vi "cameraSetup.vi"() -> ()   [LabVIEW 2024]
uses:
  <vilib>/userDefined/High Color/IMAQdx.ctl
  <vilib>/Python/Open Venv Python Session.vi
  <vilib>/vision/driver/NI_Vision_Acquisition_Software.lvlib
panel:
  out "Tracking_Err(m)":dbl=4862130.802033398
  in  "Ld(m)":dbl=5.0 format="%#_13g"
  out "GPS_Steer_CMD(Deg)":dbl=2.9943056426975447
  out "Lane":T1(graph)
  out "Third_Lane_X":dbl[](array[numeric])
  out "Third_Lane_Y":dbl[](array[numeric])
  out "Second_Lane_X":dbl[](array[numeric])
  out "Second_Lane_Y":dbl[](array[numeric])
  out "First_Lane_Y":dbl[](array[numeric])
  out "First_Lane_X":dbl[](array[numeric])
  out "ImageString":string
  out "error out":errorcluster
  out "Image":T2(plugin-control)
  in  "Test":bool=TRUE
  in  "Cam No.":T3
  out "Python Loop Process Time":u32=101
  out "Image2Array LoopTime":u32=101
  in  "stop":bool
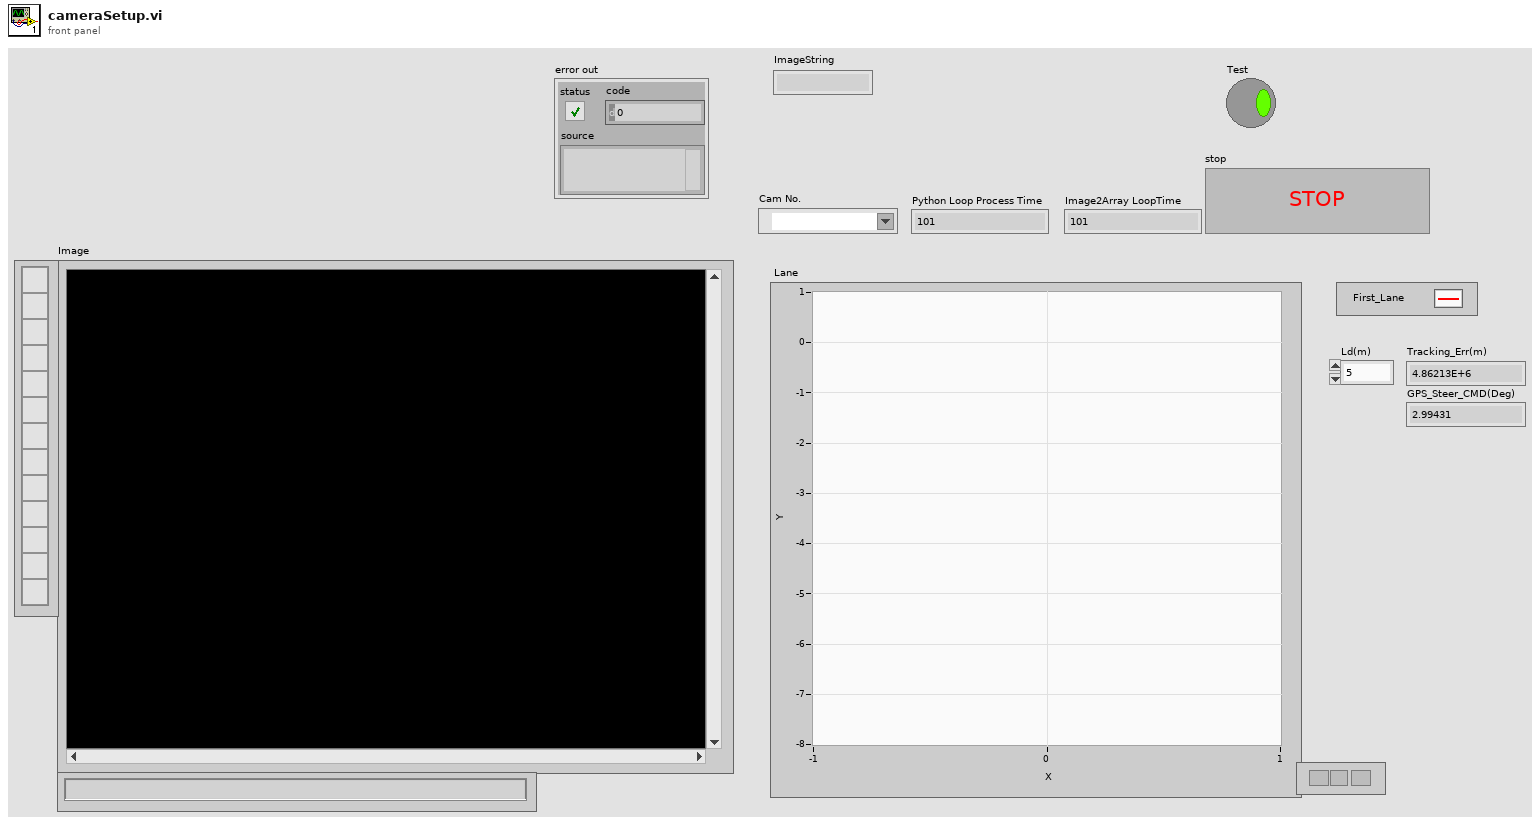
[diagram p1: front panel]
types:
  T1 = cluster{"Third_Lane_X":dbl[], "Third_Lane_Y":dbl[]}[]
  T2 = typedef "IMAQ Image.ctl" = refnum<image>
  T3 = typedef "IMAQdx.ctl" = refnum<k21>
  T4 = cluster{"First_Lane_X":dbl[], "First_Lane_Y":dbl[]}
  T5 = cluster{"Second_Lane_X":dbl[], "Second_Lane_Y":dbl[]}
  T6 = cluster{"Third_Lane_X":dbl[], "Third_Lane_Y":dbl[]}
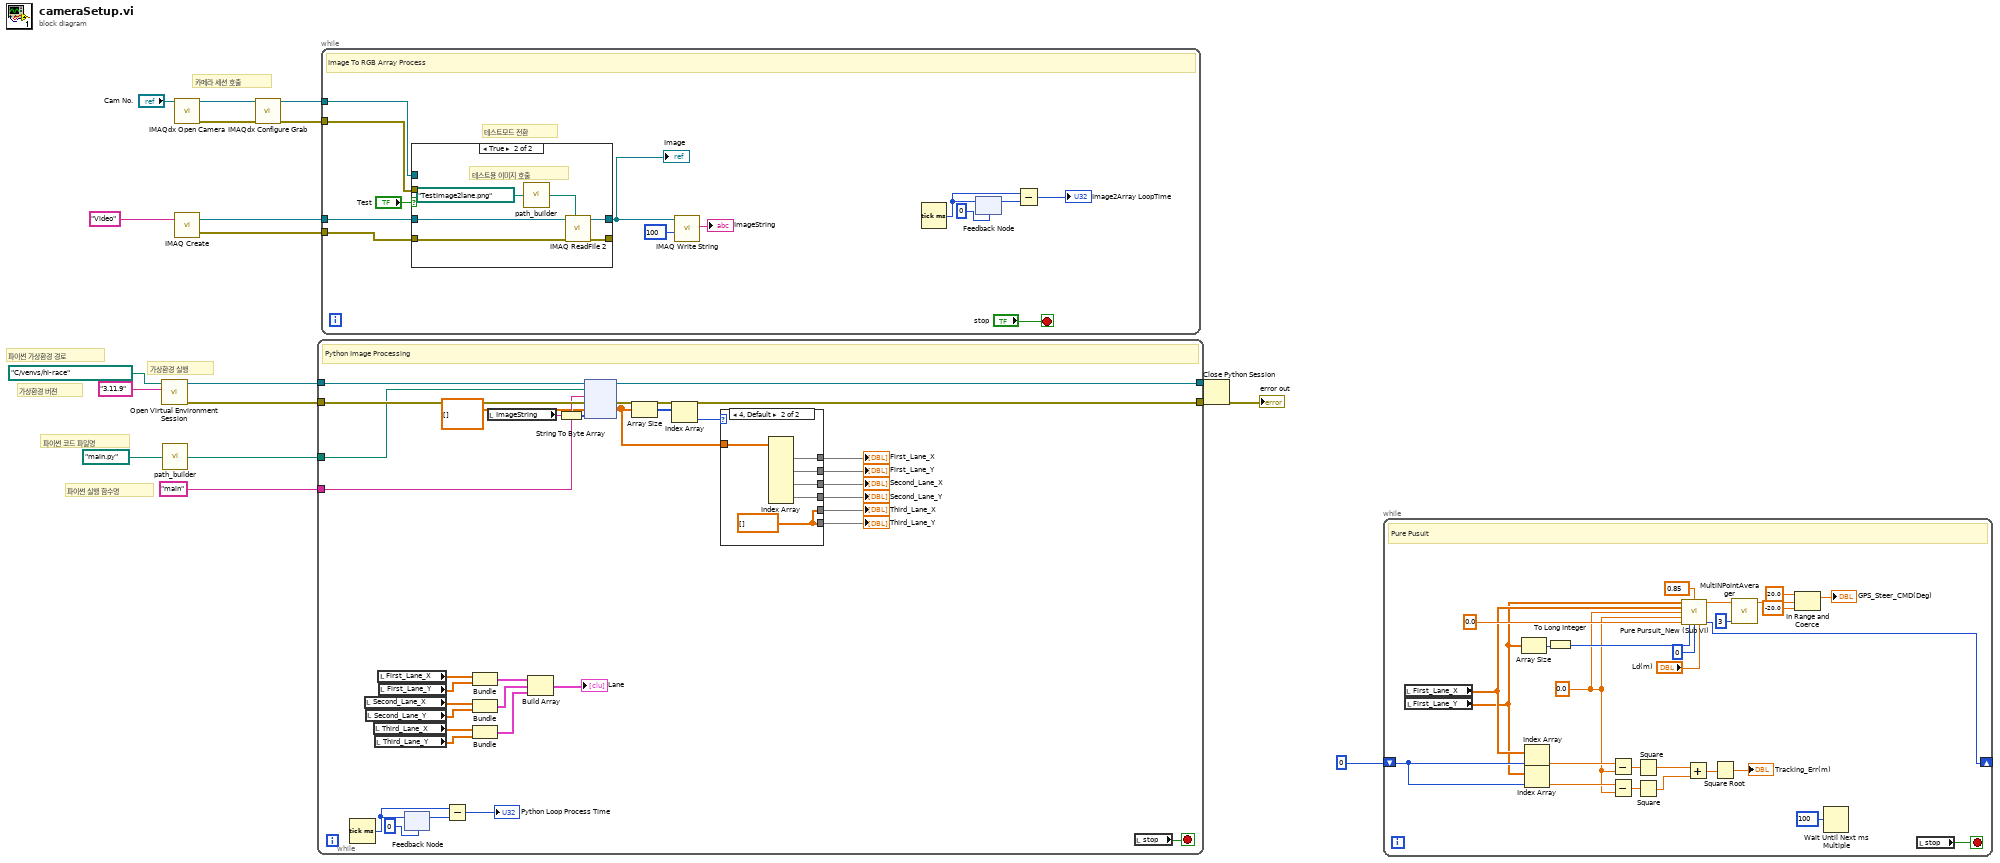
[diagram p0: block diagram]
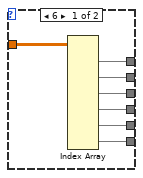
[diagram p2: hidden frame]
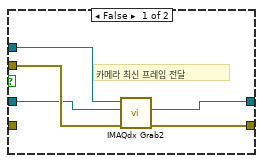
[diagram p3: hidden frame]
diagram:
  # "파이썬 실행 함수명"
  # "파이썬 코드 파일명"
  # "가상환경 실행"
  # "가상환경 버젼"
  # "파이썬 가상환경 경로"
  # "카메라 세션 호출"
  n1 = call-poly <vilib>:"Open Virtual Environment Session.vi"("Python version"="3.11.9", "Env path"=path "C:/venvs/hi-race") -> ("error out"=w11:errorcluster, "session out"=w12:refnum<k35>)  [unwired: 8 in]
  n2 = call "path_builder.vi"("Name"=path "main.py") -> ("appended path"=w10:path)
  n3 = call <vilib>:"IMAQdx Open Camera.vi"("Session In"="Cam No.") -> ("error out"=w6:errorcluster, "Session Out"=w7:T3)  [unwired: 9 in]
  n4 = call "IMAQ Create"("Image Name"="Video") -> ("New Image"=w15:T2, "error out"=w16:errorcluster)  [unwired: 4 in]
  n5 = call <vilib>:"IMAQdx Configure Grab.vi"("error in"=w6, "Session In"=w7) -> ("error out"=w3:errorcluster, "Session Out"=w4:T3)  [unwired: 8 in]
  n6 = while {
    tunnel: w10 -> [w48]
    tunnel: "main" ("module out") -> [w47]
    tunnel: w12 -> [w50]
    tunnel: [w52] -> w14
    tunnel: w11 -> [w49]
    tunnel: [w51] -> w13
    stop <- w46 stop-if-true
    # "Python Image Processing"
    n7 = Tick Count (ms)() -> (millisecond timer value=w42:u32)
    n8 = local read "Second_Lane_X"() -> (w27:dbl[])
    n9 = local read "Second_Lane_Y"() -> (w26:dbl[])
    n10 = local read "Third_Lane_X"() -> (w25:dbl[])
    n11 = local read "Third_Lane_Y"() -> (w24:dbl[])
    n12 = local read "First_Lane_X"() -> (w29:dbl[])
    n13 = local read "First_Lane_Y"() -> (w28:dbl[])
    n14 = feedback #1(u32 0 ("millisecond timer value")) -> (w43:u32)
    n15 = feedback-in #1(w42) -> ()
    n16 = Subtract(x=w42, y=w43) -> (x-y=→"Python Loop Process Time":u32)
    n17 = Bundle("First_Lane_X"=w29, "First_Lane_Y"=w28) -> (w23:T4)  [unwired: 1 in]
    n18 = Bundle("Second_Lane_X"=w27, "Second_Lane_Y"=w26) -> (w22:T5)  [unwired: 1 in]
    n19 = Bundle("Third_Lane_X"=w25, "Third_Lane_Y"=w24) -> (w21:T6)  [unwired: 1 in]
    n20 = local read "ImageString"() -> (w40:string)
    n21 = Build Array(w23, w22, w21) -> (→"Lane":T1)
    n22 = String To Byte Array(string=w40) -> (unsigned byte array=w39:u8[])
    n23 = node(w50, w48, w47, w49, dbl[][] [] ("appended array"), w39) -> (w52:refnum<k35>, w51:errorcluster, w38:dbl[][])  [unwired: 1 in, 2 out]
    n24 = Array Size(array=w38) -> (size(s)=w37:i32[])
    n25 = Index Array(array=w37) -> (element=w36:i32)  [unwired: 1 in]
    n26 = case shown="4, Default" w36 {
      tunnel: w38 -> [w59 w65]
      tunnel: [w58 w64] -> w35
      tunnel: [w57 w63] -> w34
      tunnel: [w56 w62] -> w33
      tunnel: [w55 w61] -> w32
      tunnel: [w54 w60] -> w31
      tunnel: [w53 w60] -> w30
      frame 6 {
        n27 = Index Array(array=w59) -> (element #1=w58:dbl[], element #2=w57:dbl[], element #3=w56:dbl[], element #4=w55:dbl[], element #5=w54:dbl[], element #6=w53:dbl[])  [unwired: 12 in]
      }
      frame 4, Default {
        w60 = dbl[] [] ("appended array")
        n28 = Index Array(array=w65) -> (element #1=w64:dbl[], element #2=w63:dbl[], element #3=w62:dbl[], element #4=w61:dbl[])  [unwired: 8 in]
      }
    }
    "First_Lane_X" <- w35
    "First_Lane_Y" <- w34
    "Second_Lane_X" <- w33
    "Second_Lane_Y" <- w32
    "Third_Lane_X" <- w31
    "Third_Lane_Y" <- w30
    n29 = local read "stop"() -> (w46:bool)
  }
  n30 = while {
    tunnel: w16 -> [w78]
    tunnel: w15 -> [w77]
    tunnel: w4 -> [w69]
    tunnel: w3 -> [w70]
    stop <- "stop" stop-if-true
    # "테스트모드 전환"
    # "Image To RGB Array Process"
    n31 = case shown="True" "Test" {
      tunnel: w78 -> [_ w89]
      tunnel: w77 -> [w79 w88]
      tunnel: [w80 w87] -> _
      tunnel: [w81 w86] -> w68
      tunnel: w70 -> [w83 _]
      tunnel: w69 -> [w82 _]
      frame False {
        # "카메라 최신 프레임 전달"
        n32 = call <vilib>:"IMAQdx Grab2.vi"("error in"=w83, "Image In"=w79, "Session In"=w82) -> ("error out"=w80:errorcluster, "Image Out"=w81:T2)  [unwired: 5 in, 2 out]
      }
      frame True {
        # "테스트용 이미지 호출"
        n33 = call "path_builder.vi"("Name"=path "TestImage2lane.png") -> ("appended path"=w85:path)
        n34 = call "IMAQ ReadFile 2"("File Path"=w85, "error in (no error)"=w89, "Image"=w88) -> ("error out"=w87:errorcluster, "Image Out"=w86:T2)  [unwired: 4 in, 3 out]
      }
    }
    "Image" <- w68
    n35 = call-poly "IMAQ Write String"("Image Quality"=u32 100, "Image"=w68) -> ("FileString"=→"ImageString":string)  [unwired: 7 in, 2 out]
    n36 = Tick Count (ms)() -> (millisecond timer value=w76:u32)
    n37 = feedback #2(u32 0 ("millisecond timer value")) -> (w75:u32)
    n38 = feedback-in #2(w76) -> ()
    n39 = Subtract(x=w76, y=w75) -> (x-y=→"Image2Array LoopTime":u32)
  }
  n40 = Close Python Session(session in=w14, error in=w13) -> (11:→"error out":errorcluster)
  n41 = while {
    shift-right: [w116] -> _
    shift-left: 0 ("Index(near vehicle)") -> [w115]
    stop <- w114 stop-if-true
    w90 = 0.0 ("Y_Current")
    # "Pure Pusuit"
    n42 = local read "First_Lane_X"() -> (w92:dbl[])
    n43 = local read "First_Lane_Y"() -> (w91:dbl[])
    n44 = Array Size(array=w91) -> (size(s)=w101:i32)
    n45 = Index Array(array=w92, index=w115) -> (element=w112:dbl)
    n46 = Index Array(array=w91, index=w115) -> (element=w113:dbl)
    n47 = To Long Integer(number=w101) -> (32bit integer=w100:i32)
    n48 = Subtract(x=w112, y=w90) -> (x-y=w107:dbl)
    n49 = Subtract(x=w113, y=w90) -> (x-y=w106:dbl)
    n50 = Square(x=w107) -> (x^2=w105:dbl)
    n51 = Square(x=w106) -> (x^2=w104:dbl)
    n52 = call "Pure Pursuit_New (Sub VI).vi"("x_lat_path"=w91, "L"=0.85, "y_long_path"=w92, "X_Current"=w90, "Y_Current"=w90, "Heading_Current"=0.0, "#pnt"=w100, "WP no_pre"=0, "LAD"="Ld(m)") -> ("Steer_CMD(Deg)"=w96:dbl, "Index(near vehicle)"=w116:i32)  [unwired: 3 in, 2 out]
    n53 = Add(x=w105, y=w104) -> (x+y=w103:dbl)
    n54 = Square Root(x=w103) -> (sqrt(x)=→"Tracking_Err(m)":dbl)
    n55 = call "MultiNPointAverager.vi"("N point average"=3 ("WP no_pre"), "Data_input"=w96) -> ("숫자형"=w111:dbl)  [unwired: 9 in]
    n56 = In Range and Coerce(upper limit=20.0, x=w111, lower limit=-20.0) -> (coerced(x)=→"GPS_Steer_CMD(Deg)":dbl)  [unwired: 1 out]
    n57 = Wait Until Next ms Multiple(millisecond multiple=u32 100 ("ms 배수")) -> ()  [unwired: 1 out]
    n58 = local read "stop"() -> (w114:bool)
  }
